vi "Close MeasurementLink Session.vi"(8 "error in":errorcluster, 9 "initialize and close session behavior":T1, 10 "session in":variant, 11 "session factory in":refnum<class "Session Factory.lvclass">) -> (0 "error out":errorcluster)   [LabVIEW 2020, in "MeasurementLink niFGEN.lvlib" / "Session Factory.lvclass"]
uses:
  Session Factory.lvclass
  MeasurementLink Instrument/ISession Factory/Initialize and Close Session Behavior.ctl
  Session Factory.lvclass/Session Factory.ctl
  MeasurementLink Instrument/ISession Factory/ISession Factory.lvclass
  <instrlib>/niFgen/niFgen.llb/niFgen Close.vi
  <instrlib>/niFgen/niFgen.llb/niFgen Detach gRPC Session.vi
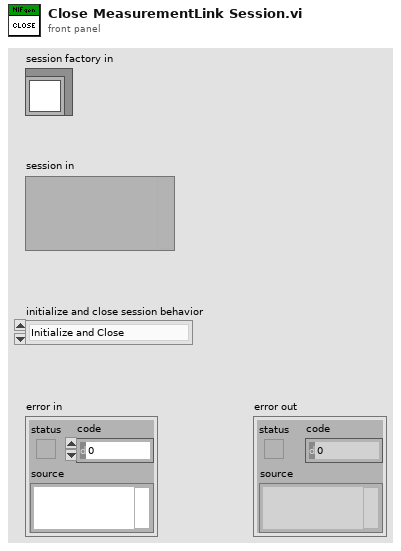
[diagram p1: front panel]
types:
  T1 = typedef "MeasurementLink Instrument.lvlib/ISession Factory.lvclass/Initialize and Close Session Behavior.ctl" = enum16{"Initialize and Close", "Attach and Detach", "Initialize and Detach", "Attach and Close"}
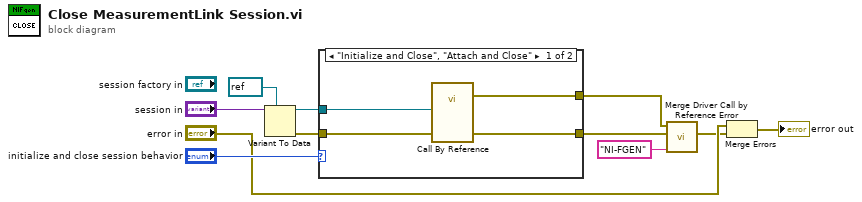
[diagram p0: block diagram]
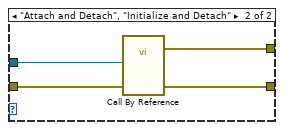
[diagram p2: hidden frame]
diagram:
  n1 = Variant To Data(type=refnum<k15> refnum ("Instrument Handle"), Variant="session in") -> (data=w7:refnum<k15>, error out=w8:errorcluster)  [unwired: 1 in]
  n2 = case shown="\"Initialize and Close\", \"Attach and Close\"" "initialize and close session behavior" {
    tunnel: w8 -> [w15 w19]
    tunnel: w7 -> [w13 w18]
    tunnel: [w14 w17] -> w3
    tunnel: [w12 w16] -> w1
    frame "Initialize and Close", "Attach and Close" {
      n3 = call-by-ref "?"("error in (no error)"=w15, "Instrument Handle"=w13) -> (error out=w12:errorcluster, 0:"error out"=w14:errorcluster)  [unwired: 11 in, 1 out]
    }
    frame "Attach and Detach", "Initialize and Detach" {
      n4 = call-by-ref "?"("error in (no error)"=w19, "Instrument Handle"=w18) -> (error out=w16:errorcluster, 0:"error out"=w17:errorcluster)  [unwired: 11 in, 1 out]
    }
  }
  n5 = call "Merge Driver Call by Reference Error.vi"("driver name"="NI-FGEN", "called vi error"=w3, "call by ref error"=w1) -> ("error out"=w2:errorcluster)  [unwired: 8 in]
  n6 = Merge Errors("error in", w2) -> (→"error out":errorcluster)
